vi "Check if NIPM is Upgadable.vi"(8 "error in (no error)":errorcluster) -> (0 "error out":errorcluster, 2 "Command line":string, 3 "Upgradable ?":bool)   [LabVIEW 2022 SP3, in "NIPM_Functions.lvlib"]
uses:
  NIPM_Functions.lvlib
  <vilib>/National Instruments/NIPM API (Beta)/NIPM_API.lvlib
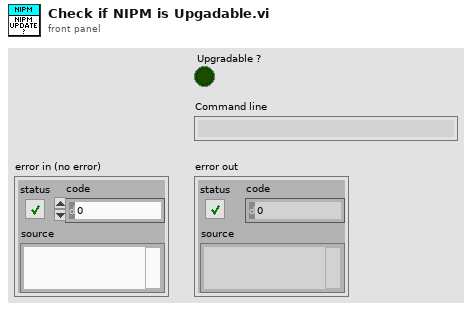
[diagram p1: front panel]
types:
  T1 = typedef "NIPM_API.lvlib/feed.ctl" = cluster{"Name":string, "URI":string}
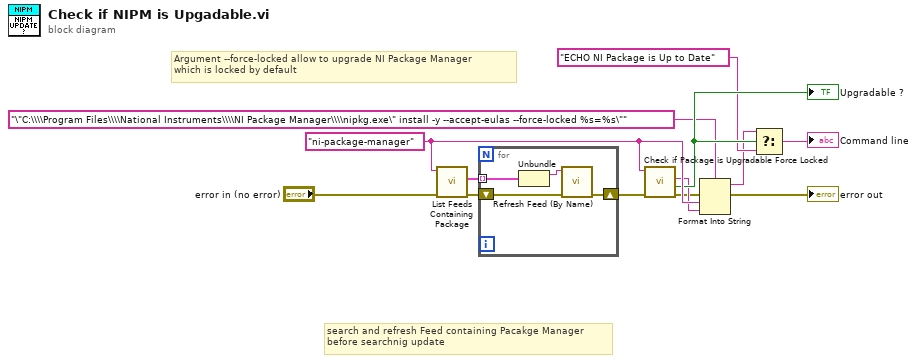
[diagram p0: block diagram]
diagram:
  w13 = "ni-package-manager" ("package name")
  # "search and refresh Feed containing Pacakge Manager \nbefore searchnig update"
  # "Argument --force-locked allow to upgrade NI Package Manager \nwhich is locked by default"
  n1 = call <vilib>:"List Feeds Containing Package.vi"("error in"="error in (no error)", "package name"=w13) -> ("error out"=w11:errorcluster, "feeds"=w10:T1[])  [unwired: 8 in]
  n2 = for {
    tunnel: w10 -> [w17] mode=indexing
    shift-right: [w15] -> w12
    shift-left: w11 -> [w16]
    n3 = Unbundle(w17) -> ("Name"=w14:string)  [unwired: 1 out]
    n4 = call <vilib>:"Refresh Feed (By Name).vi"("error in"=w16, "feed name in"=w14) -> ("error out"=w15:errorcluster)  [unwired: 8 in, 1 out]
  }
  n5 = call "Check if Package is Upgradable Force Locked.vi"("error in"=w12, "package name"=w13) -> ("error out"=w3:errorcluster, "upgradable?"=w8:bool, "version to upgrade to"=w7:string)  [unwired: 5 in, 2 out]
  "Upgradable ?" <- w8
  n6 = Format Into String(format string="\"C:\\\\Program Files\\\\National Instruments\\\\NI Package Manager\\\\nipkg.exe\" install -y --accept-eulas --force-locked %s=%s\"", error in=w3, w13, w7) -> (resulting string=w4:string, error out=→"error out":errorcluster)  [unwired: 1 in]
  n7 = Select(t=w4, s=w8, f="ECHO NI Package is Up to Date") -> (s? t:f=→"Command line":string)
